vi "Populate Tree Control Recursive Priv.vi"(4 "Show IDs (True)":bool=TRUE, 6 "Indent":i32, 7 "Data Types Dict":variant, 8 "error in":errorcluster, 9 "Items":T1(array[cluster]), 10 "Child IDs":string[](array[string]), 11 "Tree Dictionary In":variant) -> (0 "error out":errorcluster, 1 "Items Out":T1(array[cluster]), 3 "Tree Dictionary Out":variant)   [LabVIEW 2020, in "NI_VIAnCFGDataStructure.lvlib" / "Tree.lvclass"]
uses:
  <vilib>/addons/analyzer/VIAnCFGDataStructure/Tree Manager/Tree.lvclass
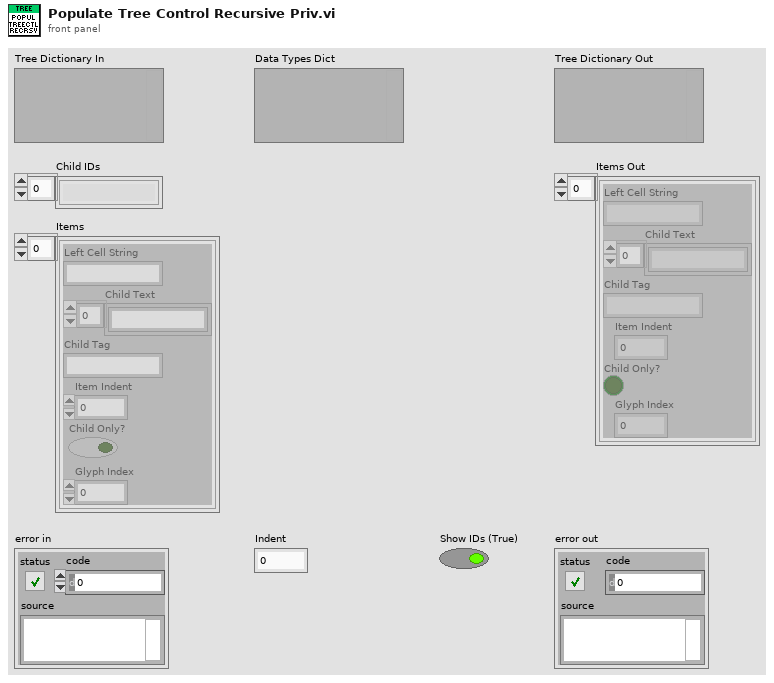
[diagram p1: front panel]
types:
  T1 = cluster{"Left Cell String":string, "Child Text":string[], "Child Tag":string, "Item Indent":i32, "Child Only?":bool, "Glyph Index":i32}[]
  T2 = cluster{"Left Cell String":string, "Child Text":string[], "Child Tag":string, "Item Indent":i32, "Child Only?":bool, "Glyph Index":i32}
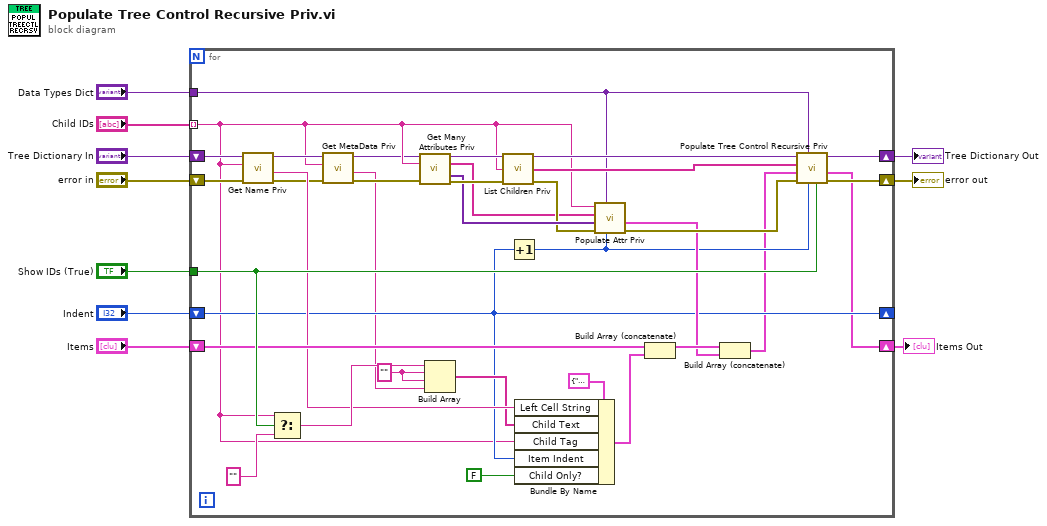
[diagram p0: block diagram]
diagram:
  n1 = for {
    tunnel: "Child IDs" -> [w16] mode=indexing
    shift-right: [w40] -> w7
    shift-left: "Tree Dictionary In" -> [w43]
    shift-right: [w38] -> w10
    shift-left: "error in" -> [w42]
    tunnel: "Show IDs (True)" -> [w34]
    tunnel: "Data Types Dict" -> [w18]
    shift-right: [w19] -> w1
    shift-left: "Items" -> [w30]
    shift-right: [w22] -> _
    shift-left: "Indent" -> [w22]
    w11 = "" ("element")
    n2 = call <vilib>:"Get Name Priv.vi"("error in"=w42, "Unique ID"=w16, "Tree Dictionary"=w43) -> ("error out"=w15:errorcluster, "Name"=w28:string, "Tree Dictionary Out"=w17:variant)  [unwired: 6 in]
    n3 = Select(t=w16, s=w34, f="") -> (s? t:f=w32:string)
    n4 = call <vilib>:"Get MetaData Priv.vi"("error in"=w15, "Unique ID"=w16, "Tree Dictionary"=w17) -> ("error out"=w13:errorcluster, "MetaData"=w12:string, "Tree Dictionary Out"=w14:variant)  [unwired: 6 in]
    n5 = call <vilib>:"Get Many Attributes Priv.vi"("Tree Dictionary In"=w14, "Unique ID"=w16, "error in"=w13) -> ("Tree Dictionary Out"=w45:variant, "Attribute Names"=w31:string[], "Attribute Values"=w36:variant[], "error out"=w44:errorcluster)  [unwired: 8 in, 1 out]
    n6 = Build Array(w32, w11, w11, w12) -> (w26:string[])
    n7 = call <vilib>:"List Children Priv.vi"("Tree Dictionary"=w45, "Parent ID"=w16, "Error In"=w44) -> ("Tree Dictionary Out"=w41:variant, "Child IDs"=w39:string[], "Error Out"=w35:errorcluster)  [unwired: 10 in]
    n8 = Increment(x=w22) -> (x+1=w21:i32)
    n9 = Bundle By Name(cluster=T2 {"Left Cell String"="", "Child Text"=[], "Child Tag"="", "Item Indent"=0, "Child Only?"=FALSE, "Glyph Index"=0} ("Item"), "Left Cell String"=w28, "Child Text"=w26, "Child Tag"=w16, "Item Indent"=w22, "Child Only?"=FALSE) -> (w25:T2)
    n10 = call <vilib>:"Populate Attr Priv.vi"("Item Indent"=w21, "Data Types Dict"=w18, "error in"=w35, "Attribute Values"=w36, "Attribute Names"=w31, "Unique ID"=w16) -> ("error out"=w37:errorcluster, "Attr Items"=w23:T1)  [unwired: 4 in]
    n11 = Build Array (concatenate)(w30, w25) -> (w24:T1)
    n12 = Build Array (concatenate)(w24, w23) -> (w20:T1)
    n13 = call <vilib>:"Populate Tree Control Recursive Priv.vi"("Show IDs (True)"=w34, "Indent"=w21, "Data Types Dict"=w18, "error in"=w37, "Items"=w20, "Child IDs"=w39, "Tree Dictionary In"=w41) -> ("error out"=w38:errorcluster, "Items Out"=w19:T1, "Tree Dictionary Out"=w40:variant)  [unwired: 2 in]
  }
  "error out" <- w10
  "Tree Dictionary Out" <- w7
  "Items Out" <- w1
